vi "CT_DelayTL_to_QSW.vi"(0 "Very Fast Timing In":dbl[](array[slide])=[1100.0, 3200.0, 3254.0, 3290.0, 3100.0, 3080.0, 0.0, 3100.0] min=0.0 max=4000.0 step=2.0 scale=0.0..4000.0 scale format="%#_3f", 1 "TL Index":i32=5, 2 "Ultra Fast Timing":dbl[](array[slide])=[180.0, 95.0, 0.0] min=0.0 max=1000.0 step=1.0 scale=0.0..1000.0 scale format="%#_3f", 3 "Holdoff Guess (us)":u32, 4 "TS Ref Shot":bool, 5 "Size of Trig Waveform":dbl=4000.0, 6 "QSW Index":i32=1, 7 "Form Index":i32=1) -> (8 "Very Fast Timing Out":dbl[](array[slide])=[1100.0, 3200.0, 3254.0, 3290.0, 3100.0, 3080.0, 0.0, 3100.0] min=0.0 max=4000.0 step=2.0 scale=0.0..4000.0 scale format="%#_3f")   [LabVIEW 2016]
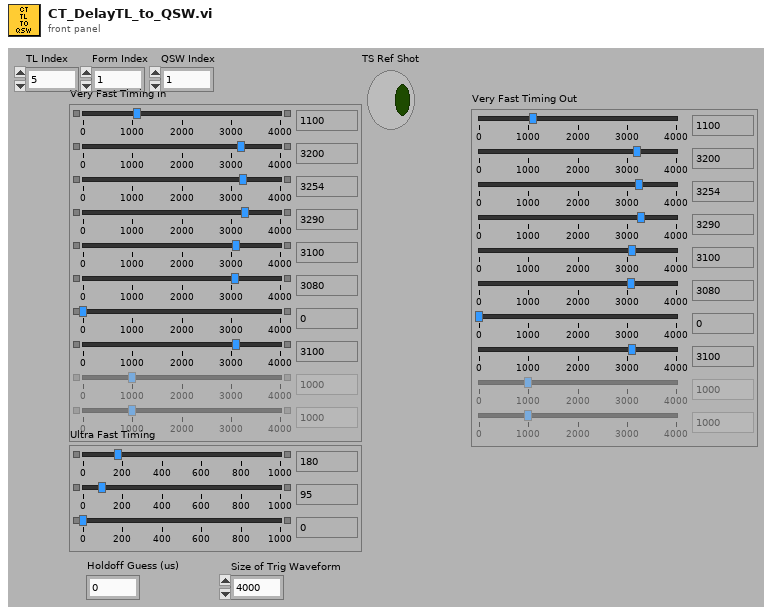
[diagram p1: front panel]
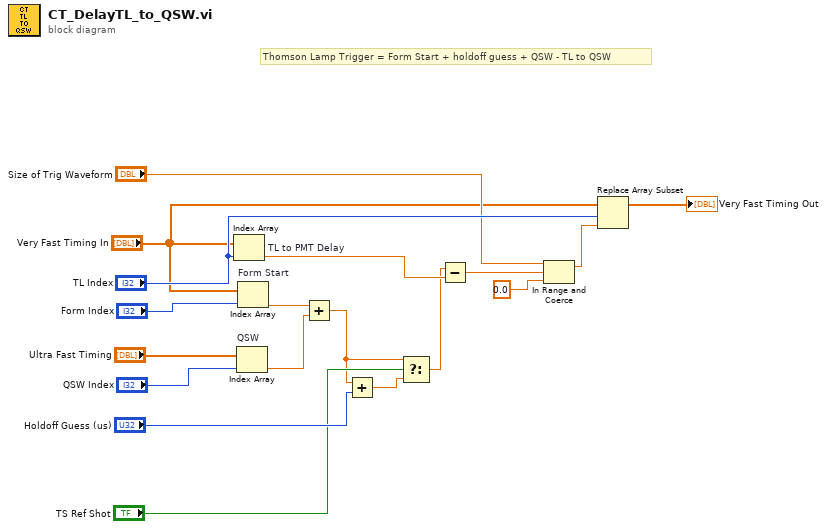
[diagram p0: block diagram]
diagram:
  # "Thomson Lamp Trigger = Form Start + holdoff guess + QSW - TL to QSW"
  n1 = Index Array "TL to PMT Delay"(array="Very Fast Timing In", index="TL Index") -> (element=w5:dbl)
  n2 = Index Array "QSW"(array="Ultra Fast Timing", index="QSW Index") -> (element=w7:dbl)
  n3 = Index Array "Form Start"(array="Very Fast Timing In", index="Form Index") -> (element=w8:dbl)
  n4 = Add(x=w8, y=w7) -> (x+y=w3:dbl)
  n5 = Add(x=w3, y="Holdoff Guess (us)") -> (x+y=w1:dbl)
  n6 = Select(t=w3, s="TS Ref Shot", f=w1) -> (s? t:f=w2:dbl)
  n7 = Subtract(x=w2, y=w5) -> (x-y=w15:dbl)
  n8 = In Range and Coerce(upper limit="Size of Trig Waveform", x=w15, lower limit=0.0) -> (coerced(x)=w14:dbl)  [unwired: 1 out]
  n9 = Replace Array Subset(array="Very Fast Timing In", new element=w14, index="TL Index") -> (→"Very Fast Timing Out":dbl[])
